vi "add to build spec.vi"(8 "error in (no error)":errorcluster, 11 "PackedLibrary in":refnum<class "PackedLibrary.lvclass">) -> (0 "error out":errorcluster, 3 "PackedLibrary out":refnum<class "PackedLibrary.lvclass">)   [LabVIEW 2024, in "PackedLibrary.lvclass"]
uses:
  PackedLibrary.lvclass
  PackedLibrary.lvclass/PackedLibrary.ctl
  D:/_repos/sandbox/github_p/labview-tools/cicd_tools/src/builders/parent/Builder.lvclass
  D:/_repos/sandbox/github_p/labview-tools/cicd_tools/src/builders/packed_library/PackedLibrary.lvclass
  parent/Builder.lvclass
  <vilib>/AppBuilder/AB_API/PPL/NI_AB_API_PPL.lvclass
  C:/Program Files/National Instruments/LabVIEW 2024/vi.lib/AppBuilder/AB_API/Targetfile/NI_AB_API_Targetfile.lvclass
  C:/Program Files/National Instruments/LabVIEW 2024/vi.lib/AppBuilder/AB_API/Build/NI_AB_API_Build.lvclass
  C:/Program Files/National Instruments/LabVIEW 2024/vi.lib/AppBuilder/AB_API/PPL/NI_AB_API_PPL.lvclass
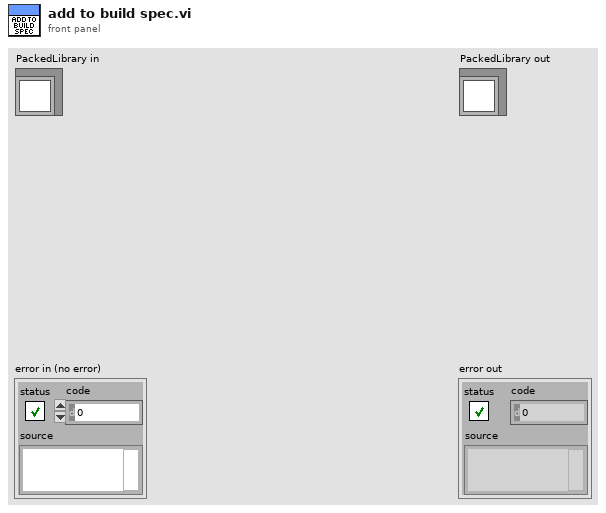
[diagram p1: front panel]
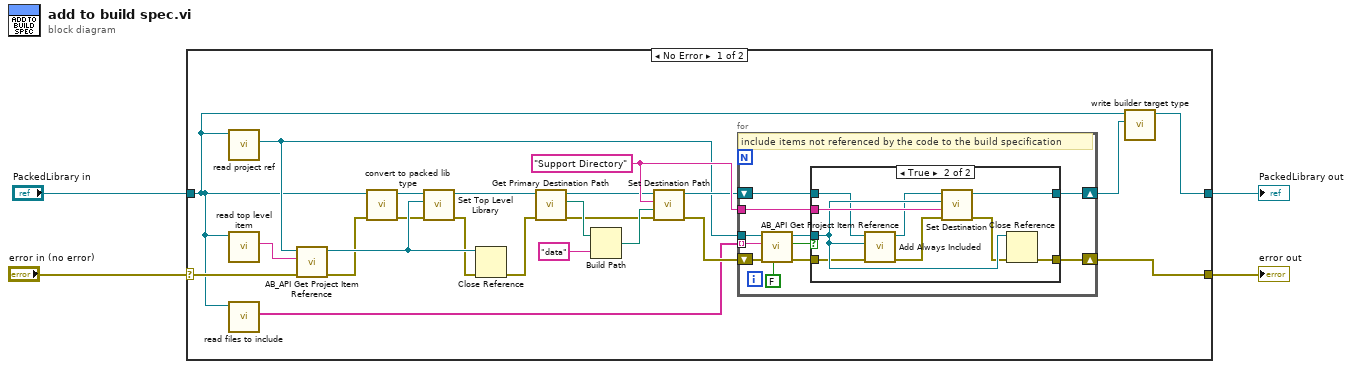
[diagram p0: block diagram]
diagram:
  n1 = case shown="No Error" "error in (no error)" {
    selector: "error in (no error)" -> [w27 w51]
    tunnel: "PackedLibrary in" -> [w6 w50]
    tunnel: [w24 w51] -> w2
    tunnel: [w5 w50] -> w1
    frame No Error {
      w25 = "Support Directory" ("Destination label")
      n2 = call "read project ref.vi"("Builders in"=w6) -> ("project ref"=w10:refnum<vi>)  [unwired: 10 in]
      n3 = call "read top level item.vi"("Builder in"=w6) -> ("top level item"=w8:string)  [unwired: 10 in]
      n4 = call "read files to include.vi"("Builder in"=w6) -> ("files to include"=w9:string[])  [unwired: 10 in]
      n5 = call <vilib>:"AB_API Get Project Item Reference.vi"("error in (no error)"=w27, "Name"=w8, "Project Refnum"=w10) -> ("error out"=w14:errorcluster, "ProjectItem Refnum"=w16:refnum<vi>)  [unwired: 6 in, 1 out]
      n6 = call "convert to packed lib type.vi"("error in (no error)"=w14, "PackedLibrary in"=w6) -> ("error out"=w12:errorcluster, "NI_AB_API_PPL out"=w11:refnum<class "NI_AB_API_PPL.lvclass">)  [unwired: 8 in]
      n7 = call-dynamic "Set Top Level Library.vi"("error in (no error)"=w12, "ProjectItem Refnum"=w16, "PPL in"=w11) -> ("error out"=w15:errorcluster, "PPL out"=w13:refnum<class "NI_AB_API_PPL.lvclass">)  [unwired: 7 in]
      n8 = Close Reference(reference=w16, error in (no error)=w15) -> (error out=w17:errorcluster)
      n9 = call-dynamic "Get Primary Destination Path.vi"("error in (no error)"=w17, "PPL in"=w13) -> ("error out"=w21:errorcluster, "Primary destination path"=w22:path, "PPL out"=w20:refnum<class "NI_AB_API_PPL.lvclass">)  [unwired: 7 in]
      n10 = Build Path(base path=w22, name or relative path="data" ("Destination label")) -> (appended path=w23:path)
      n11 = call-dynamic "Set Destination Path.vi"("error in (no error)"=w21, "Destination path"=w23, "Destination label"=w25, "PPL in"=w20) -> ("error out"=w18:errorcluster, "PPL out"=w19:refnum<class "NI_AB_API_PPL.lvclass">)  [unwired: 6 in]
      n12 = for {
        tunnel: w10 -> [w34]
        tunnel: w9 -> [w33] mode=indexing
        shift-right: [w35] -> w24
        shift-left: w18 -> [w38]
        shift-right: [w36] -> w7
        shift-left: w19 -> [w32]
        tunnel: w25 -> [w28]
        # "include items not referenced by the code to the build specification"
        n13 = call <vilib>:"AB_API Get Project Item Reference.vi"("Exclude dependencies"=FALSE, "error in (no error)"=w38, "Name"=w33, "Project Refnum"=w34) -> ("error out"=w37:errorcluster, "found?"=w30:bool, "ProjectItem Refnum"=w31:refnum<vi>)  [unwired: 5 in]
        n14 = case shown="True" w30 {
          tunnel: w37 -> [w39 w41]
          tunnel: [w40 w42] -> w36
          tunnel: [w39 w49] -> w35
          tunnel: w32 -> [w40 w45]
          tunnel: w31 -> [_ w47]
          tunnel: w28 -> [_ w48]
          frame False {
          }
          frame True {
            n15 = call-dynamic "Add Always Included.vi"("error in (no error)"=w41, "ProjectItem Refnum"=w47, "PPL in"=w45) -> ("error out"=w44:errorcluster, "PPL out"=w46:refnum<class "NI_AB_API_PPL.lvclass">)  [unwired: 7 in]
            n16 = call-dynamic "Set Destination.vi"("error in (no error)"=w44, "Destination label"=w48, "ProjectItem Refnum"=w47, "DLL in"=w46) -> ("error out"=w43:errorcluster, "DLL out"=w42:refnum<class "NI_AB_API_PPL.lvclass">)  [unwired: 6 in]
            n17 = Close Reference(reference=w47, error in (no error)=w43) -> (error out=w49:errorcluster)
          }
        }
      }
      n18 = call "write builder target type.vi"("builder target type"=w7, "Builder in"=w6) -> ("Builder out"=w5:refnum<class "PackedLibrary.lvclass">)  [unwired: 9 in]
    }
    frame Error {
    }
  }
  "error out" <- w2
  "PackedLibrary out" <- w1
